vi "Actor Core.vi"(8 "error in":errorcluster, 11 "Hardware in":refnum<class "scan_panel.lvclass">) -> (0 "error out":errorcluster, 3 "Actor out":refnum<class "Actor.lvclass">)   [LabVIEW 2015, in "scan_panel.lvclass"]
doc: "(<B>Filename</B>: Actor Framework.lvlib:Actor.lvclass:Actor Core.vi)\n\nReceives messages to the actor, reacts to them, and initiates any error handling that may shut the actor down.\n\nDescendant classes may override this VI to append parallel tasks for the actor to complete while it handles messages. Overrides use the Call Parent Method node."
uses:
  scan_panel.lvclass
  <vilib>/ActorFramework/Actor/Actor.lvclass
  scan_unit.ctl
  scan_record.ctl
  UI/panel_class/panel.lvclass/panel.ctl
  scan_settings.ctl
  <vilib>/ActorFramework/Actor/Actor.lvclass/Actor.ctl
  <vilib>/ActorFramework/Message Enqueuer/Message Enqueuer.lvclass/Message Enqueuer.ctl
  scan_panel Messages/scan_perform_scan Msg/scan_perform_scan Msg.lvclass/scan_perform_scan Msg.ctl
  <vilib>/ActorFramework/Message Enqueuer/Init from Existing Queue.vi
  <vilib>/ActorFramework/Message Enqueuer/Enqueue.vi
  <vilib>/ActorFramework/Message Priority Queue/Priority Enqueue.vi
  <vilib>/ActorFramework/Message Enqueuer/Message Enqueuer.lvclass
  scan_panel Messages/scan_perform_scan Msg/scan_perform_scan Msg.lvclass
  UI/panel_class/panel.lvclass
panel:
  in  "Notes":string
  in  "copy_bounds":bool
  in  "scan":bool
  in  "Dwell Time (s)":dbl=0.1 min=0.02
  in  "Record Type":T1=enum."None"
  in  "Save Path":path
  out "Status":string
  in  "Stage Speed":dbl=1.0
  in  "Stage Number":enum16{"1", "2"}(ring)
  in  "Unit":T2
  in  "Steps":dbl
  in  "Range [--|--]":dbl
  in  "Center Pos. (mm)":dbl
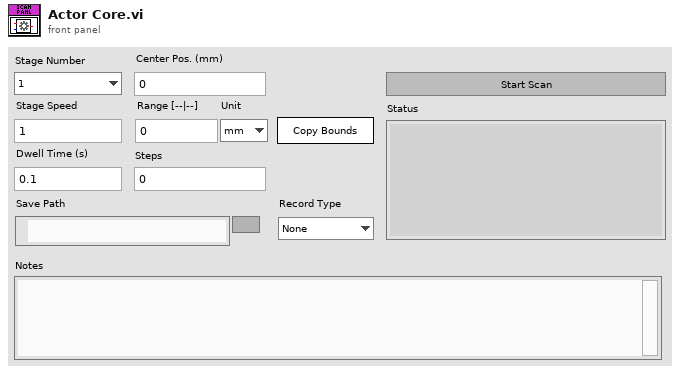
[diagram p1: front panel]
types:
  T1 = typedef "scan_record.ctl" = enum16{"hdf5", "legacy", "None"}
  T2 = typedef "scan_unit.ctl" = enum16{"mm", "s", "ms", "us", "ns", "ps", "fs"}
  T3 = cluster{"stop_ui_ref":refnum<event-registration>, "update_status":refnum<event-registration>}
  T4 = typedef "scan_settings.ctl" = cluster{"Center Pos. (mm)":dbl, "Range [--|--]":dbl, "Unit":T2, "Steps":dbl, "Stage Number":enum16{"1", "2"}, "Stage Speed":dbl, "Dwell Time (s)":dbl, "Record Type":T1, "Save Path":path, "Notes":string}
  T5 = typedef "ui_plot_references.ctl" = cluster{"plots":refnum<vi>, "chart":refnum<vi>, "graph":refnum<vi>, "map":refnum<vi>, "XY Graph":refnum<vi>}
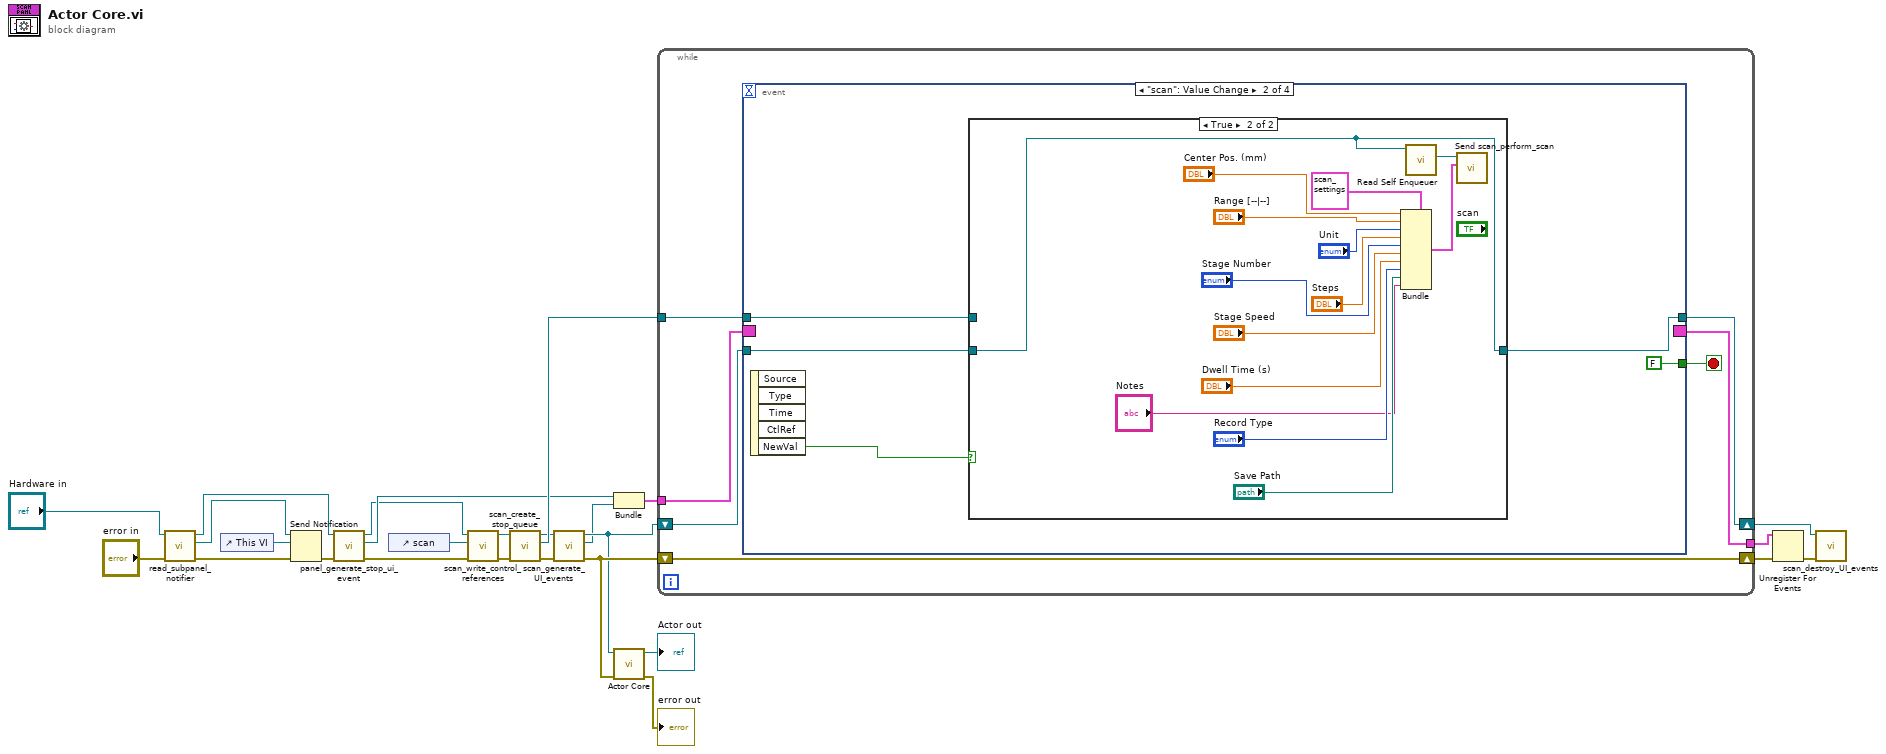
[diagram p0: block diagram]
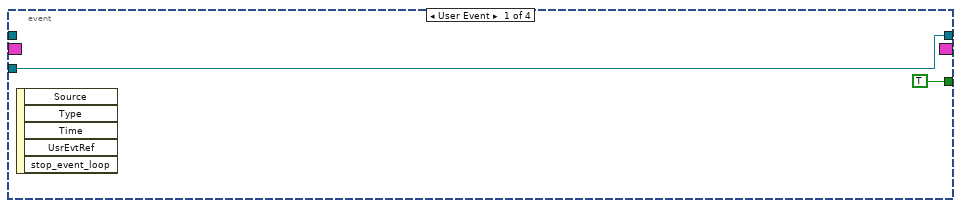
[diagram p2: hidden frame]
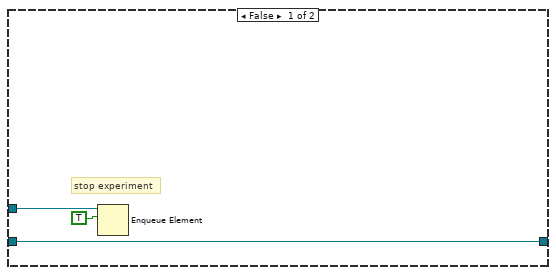
[diagram p3: hidden frame]
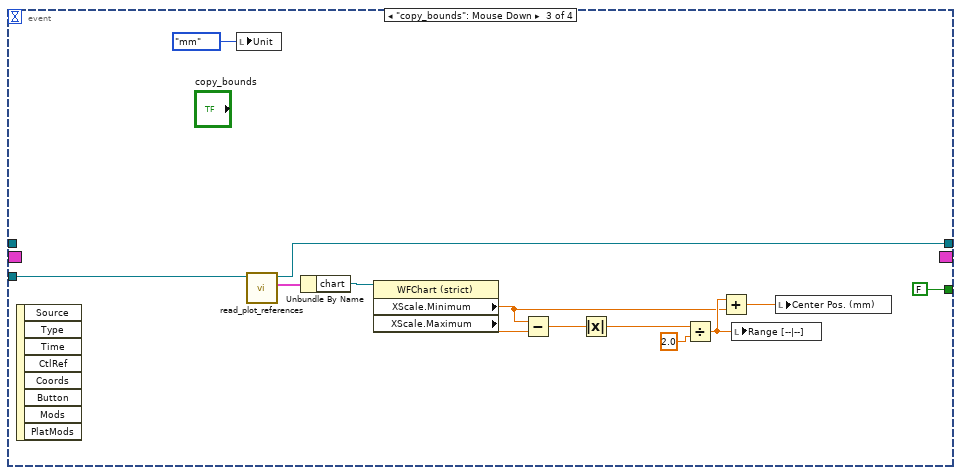
[diagram p4: hidden frame]
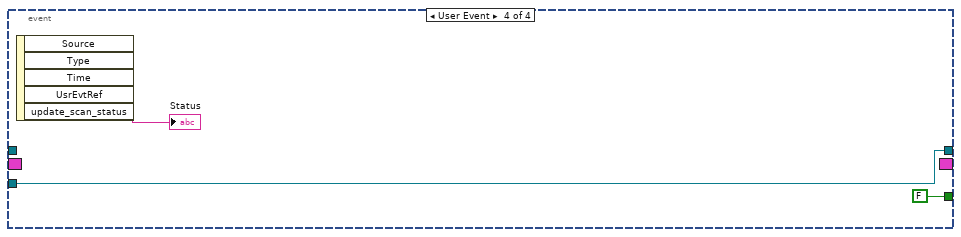
[diagram p5: hidden frame]
diagram:
  n1 = call "read_subpanel_notifier.vi"("error in (no error)"="error in", "panel in"="Hardware in") -> ("error out"=w20:errorcluster, "subpanel_notifier"=w22:refnum<notifier>, "panel out"=w21:refnum<class "scan_panel.lvclass">)  [unwired: 7 in]
  n2 = control-ref of="This VI"() -> (w24:refnum<vi>)
  n3 = Send Notification(notification=w24, notifier=w22, error in (no error)=w20) -> (error out=w19:errorcluster)  [unwired: 1 out]
  n4 = call "panel_generate_stop_ui_event.vi"("error in (no error)"=w19, "panel in"=w21) -> ("error out"=w5:errorcluster, "stop_ui_ref"=w11:refnum<event-registration>, "panel out"=w3:refnum<class "scan_panel.lvclass">)  [unwired: 7 in]
  n5 = control-ref of="scan"() -> (w1:refnum<vi>)
  n6 = call "scan_write_control_references.vi"("error in (no error)"=w5, "scan"=w1, "scan_panel in"=w3) -> ("error out"=w4:errorcluster, "scan_panel out"=w2:refnum<class "scan_panel.lvclass">)  [unwired: 7 in]
  n7 = call "scan_create_stop_queue.vi"("error in (no error)"=w4, "scan_panel in"=w2) -> ("error out"=w15:errorcluster, "stop_queue"=w16:refnum<queue>, "scan_panel out"=w13:refnum<class "scan_panel.lvclass">)  [unwired: 7 in]
  n8 = call "scan_generate_UI_events.vi"("error in (no error)"=w15, "scan_panel in"=w13) -> ("error out"=w14:errorcluster, "update_status"=w10:refnum<event-registration>, "scan_panel out"=w12:refnum<class "scan_panel.lvclass">)  [unwired: 7 in]
  n9 = Bundle("stop_ui_ref"=w11, "update_status"=w10) -> (w9:T3)  [unwired: 1 in]
  n10 = call-parent "Actor Core.vi"("error in"=w14, "Actor in"=w12) -> ("error out"=→"error out":errorcluster, "Actor out"=→"Actor out":refnum<class "Actor.lvclass">)  [unwired: 8 in]
  n11 = while {
    tunnel: w9 -> [w33]
    tunnel: [w31] -> w17
    shift-right: [w30] -> w8
    shift-left: w14 -> [w30]
    tunnel: w16 -> [w29]
    shift-right: [w27] -> w7
    shift-left: w12 -> [w28]
    stop <- w32 stop-if-true
    n12 = event shown="[1] \"scan\": Value Change" {
      selector: w33 -> [_ _ _ _]
      dyn-events: [_ _ _ _] -> w31
      timeout: _ -> [_ _ _ _]
      tunnel: [TRUE FALSE FALSE FALSE] -> w32
      tunnel: w29 -> [_ w38 _ _]
      tunnel: w28 -> [w34 w37 w70 w71]
      tunnel: [w34 w36 w59 w71] -> w27
      event User Event {
        n13 = event-data() -> ()  [unwired: 1 in, 5 out]
      }
      event "scan": Value Change {
        n14 = event-data() -> ("NewVal"=w39:bool)  [unwired: 1 in, 4 out]
        n15 = case shown="True" w39 {
          tunnel: w38 -> [w43 _]
          tunnel: w37 -> [w41 w47]
          tunnel: [w41 w47] -> w36
          frame False {
            # "stop experiment"
            n16 = Enqueue Element(queue=w43, element=TRUE) -> ()  [unwired: 2 in, 3 out]
          }
          frame True {
            n17 = Bundle(cluster=T4 {"Center Pos. (mm)"=0.0, "Range [--|--]"=0.0, "Unit"=enum."mm", "Steps"=0.0, "Stage Number"=enum."1", "Stage Speed"=1.0, "Dwell Time (s)"=0.1, "Record Type"=enum."hdf5", "Save Path"=path "", "Notes"=""} ("output cluster"), "Center Pos. (mm)"="Center Pos. (mm)", "Range [--|--]"="Range [--|--]", "Unit"="Unit", "Steps"="Steps", "Stage Number"="Stage Number", "Stage Speed"="Stage Speed", "Dwell Time (s)"="Dwell Time (s)", "Record Type"="Record Type", "Save Path"="Save Path", "Notes"="Notes") -> (w45:T4)
            n18 = call <vilib>:"Read Self Enqueuer.vi"("Actor"=w47) -> ("Self Enqueuer"=w46:refnum<class "Message Enqueuer.lvclass">)  [unwired: 10 in]
            n19 = call "Send scan_perform_scan.vi"("scan_settings"=w45, "Message Enqueuer"=w46) -> ()  [unwired: 8 in, 2 out]
          }
        }
      }
      event "copy_bounds": Mouse Down {
        n20 = event-data() -> ()  [unwired: 1 in, 8 out]
        n21 = local write "Unit"(scan_unit."mm" ("Unit")) -> ()
        n22 = call "read_plot_references.vi"("panel in"=w70) -> ("plot_references"=w69:T5, "panel out"=w59:refnum<class "scan_panel.lvclass">)  [unwired: 8 in, 1 out]
        n23 = Unbundle By Name(w69) -> ("chart"=w68:refnum<vi>)
        n24 = property class="WFChart (strict)"(reference=w68) -> ("XScale.Minimum"=w61:dbl, "XScale.Maximum"=w67:dbl)  [unwired: 1 in, 2 out]
        n25 = Subtract(x=w61, y=w67) -> (x-y=w66:dbl)
        n26 = Absolute Value(x=w66) -> (abs(x)=w65:dbl)
        n27 = Divide(x=w65, y=2.0) -> (x/y=w62:dbl)
        n28 = Add(x=w62, y=w61) -> (x+y=w60:dbl)
        n29 = local write "Range [--|--]"(w62) -> ()
        n30 = local write "Center Pos. (mm)"(w60) -> ()
      }
      event User Event {
        n31 = event-data() -> ("update_scan_status"=→"Status":string)  [unwired: 1 in, 4 out]
      }
    }
  }
  n32 = Unregister For Events(event registration refnum=w17, error in=w8) -> (error out=w6:errorcluster)
  n33 = call "scan_destroy_UI_events.vi"("error in (no error)"=w6, "scan_panel in"=w7) -> ()  [unwired: 8 in, 2 out]
